vi "Update Vibs.vi"(8 "error in":errorcluster, 11 "Accel":T1) -> (0 "error out":errorcluster)   [LabVIEW 2018, in "UDP Writer.lvlib"]
doc: "This subVI enqueues the named action in to the communications queue along with the input data."
uses:
  UDP Writer.lvlib
  Private Controls/Module Data.ctl
  Private Controls/Module Action.ctl
  27e89eef-41d2-46aa-8cf3-f2635fb257db.vi
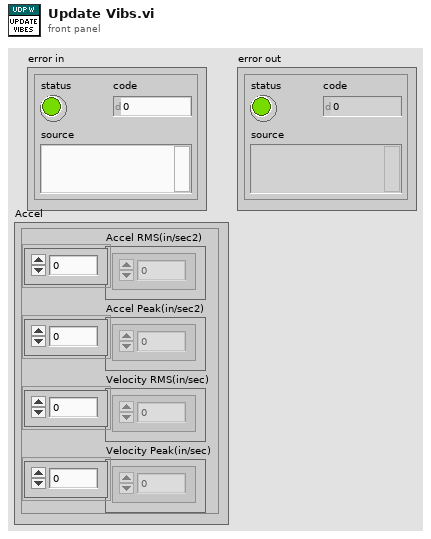
[diagram p1: front panel]
types:
  T1 = cluster{"Accel RMS(in/sec2)":dbl[], "Accel Peak(in/sec2)":dbl[], "Velocity RMS(in/sec)":dbl[], "Velocity Peak(in/sec)":dbl[]}
  T2 = typedef "UDP Writer.lvlib/Module Data.ctl" = cluster{"Data":variant, "Action":T3}
  T3 = typedef "UDP Writer.lvlib/Module Action.ctl" = enum16{"Init", "Update ARINC", "Update Waterfall", "Update RPMs", "Update Temps", "Update Modbus", "Update AI", "Update Vibs", "Write", "Error"}
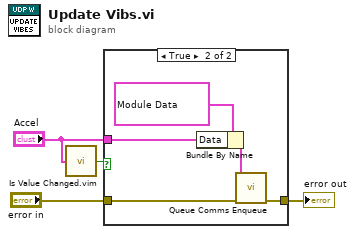
[diagram p0: block diagram]
diagram:
  n1 = call "Is Value Changed.vim"("value"="Accel") -> ("changed or first call?"=w1:bool)
  n2 = case shown="True" w1 {
    tunnel: [w5 w10] -> w4
    tunnel: "error in" -> [w5 w9]
    tunnel: "Accel" -> [_ w6]
    frame False {
    }
    frame True {
      n3 = Bundle By Name(cluster=T2 {"Data"=variant, "Action"=enum."Update Vibs"} ("element"), "Data"=w6) -> (w7:T2)
      n4 = call "Queue Comms Enqueue.vi"("error in (no error)"=w9, "element"=w7) -> ("error out"=w10:errorcluster)  [unwired: 9 in]
    }
  }
  "error out" <- w4
